vi "Log Data.vi"(0 "Test Inputs":T2 {"Nominal Output Voltage in V" format="%#.5g"; "Load Current in A" format="%#.5g"}, 5 "Test Results":T1 {"Line Regulation in %" format="%#.5g"; "Input Voltage in V" format="%#.5g"; "Input Current in A" format="%#.5g"; "Load Current in A" format="%#.5g"; "Line Regulation in %/V" format="%#.3g"; "Output Voltage in V" format="%#.5g"}, 7 "DataLogger File Path":path, 11 "error in (no error)":errorcluster) -> (15 "error out":errorcluster)   [LabVIEW 2020, in "LDO Line Regulation.lvlib"]
uses:
  LDO Line Regulation.lvlib
  Typedefs/Test Inputs.ctl
  Typedefs/Advance Settings.ctl
  Reusables/Instrument APIs/Load Output Function.ctl
  Typedefs/Test Results.ctl
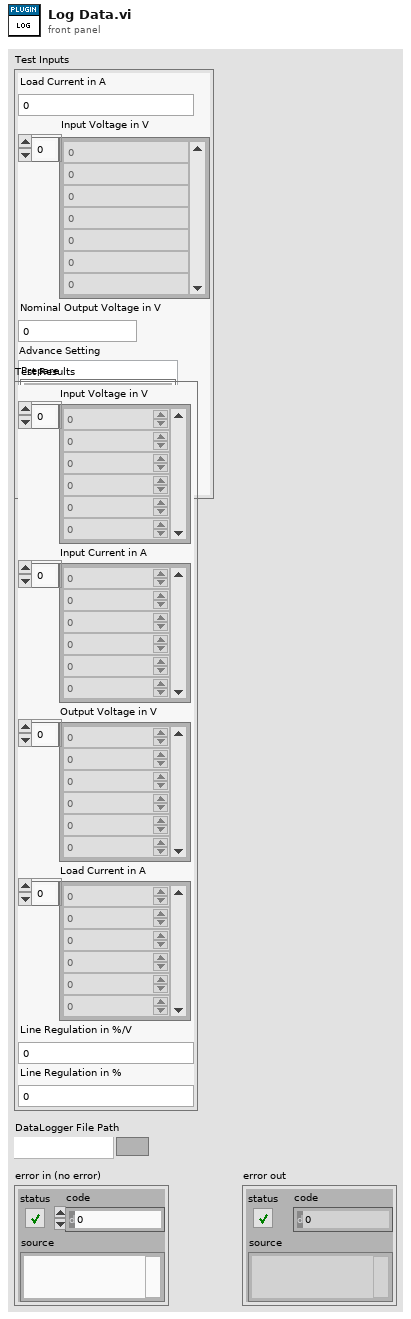
[diagram p1: front panel]
types:
  T1 = typedef "LDO Line Regulation.lvlib/Test Results.ctl" = cluster{"Input Voltage in V":dbl[], "Input Current in A":dbl[], "Output Voltage in V":dbl[], "Load Current in A":dbl[], "Line Regulation in %/V":dbl, "Line Regulation in %":dbl}
  T2 = typedef "LDO Line Regulation.lvlib/Test Inputs.ctl" = cluster{"Load Current in A":dbl, "Input Voltage in V":dbl[], "Nominal Output Voltage in V":dbl, "Advance Setting":T3}
  T3 = typedef "LDO Line Regulation.lvlib/Advance Settings.ctl" = cluster{"Prepare":cluster{"Load SMU Output Function":T4}, "Stimulus And Measure":cluster{"Loop Delay in milliSecond":u32}}
  T4 = typedef "Load Output Function.ctl" = enum16{"VoltageSource", "CurrentSource"}
  T5 = enum16{"open", "replace", "create", "open or create", "replace or create", "replace or create with confirmation"}
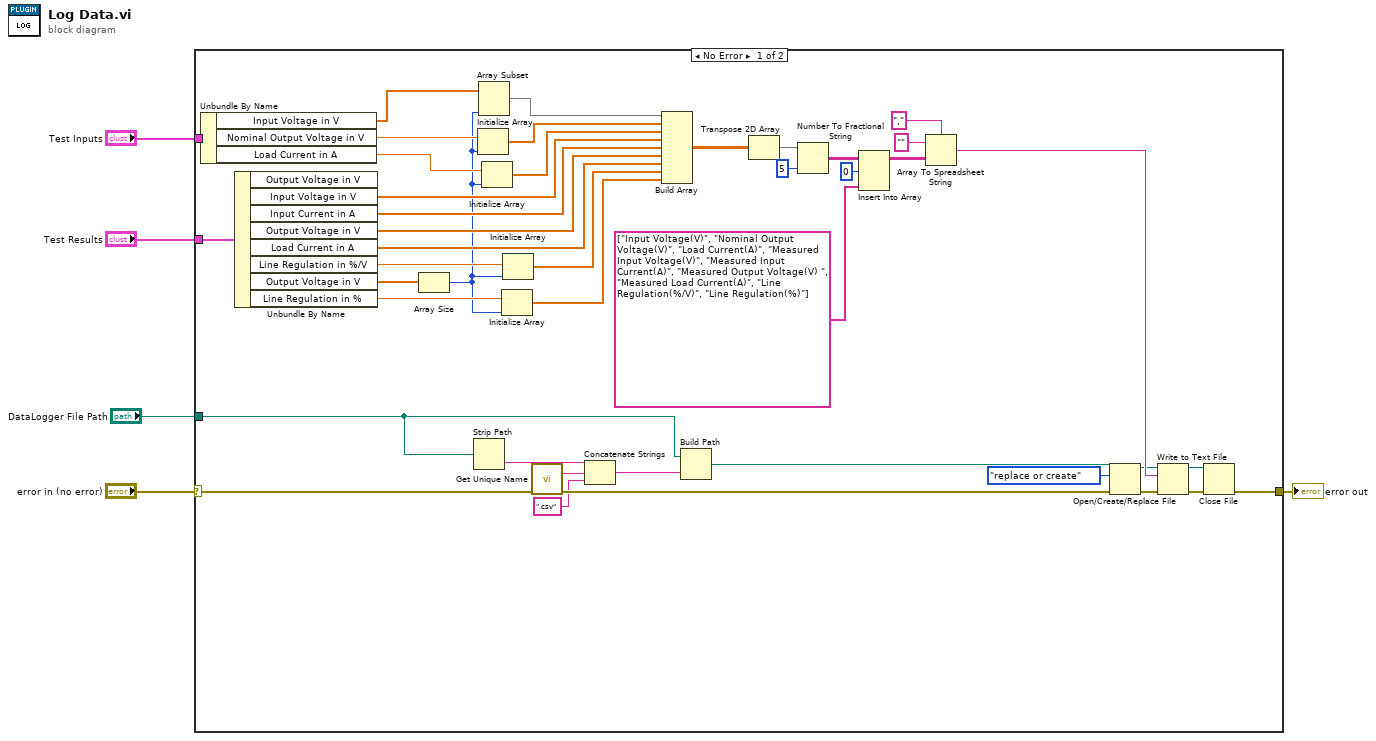
[diagram p0: block diagram]
diagram:
  n1 = case shown="No Error" "error in (no error)" {
    selector: "error in (no error)" -> [w22 w47]
    tunnel: [w30 w47] -> w4
    tunnel: "Test Inputs" -> [w46 _]
    tunnel: "Test Results" -> [w45 _]
    tunnel: "DataLogger File Path" -> [w10 _]
    frame No Error {
      n2 = Unbundle By Name(w46) -> ("Input Voltage in V"=w25:dbl[], "Nominal Output Voltage in V"=w35:dbl, "Load Current in A"=w21:dbl)
      n3 = Unbundle By Name(w45) -> ("Input Voltage in V"=w40:dbl[], "Input Current in A"=w41:dbl[], "Output Voltage in V"=w42:dbl[], "Load Current in A"=w43:dbl[], "Line Regulation in %/V"=w33:dbl, "Output Voltage in V"=w31:dbl[], "Line Regulation in %"=w8:dbl)  [unwired: 1 out]
      n4 = Array Size(array=w31) -> (size(s)=w7:i32)
      n5 = Strip Path(path=w10) -> (name=w13:string)  [unwired: 1 out]
      n6 = Initialize Array(w35, w7) -> (w34:dbl[])
      n7 = Array Subset(array=w25, length=w7) -> (w24:dbl[])  [unwired: 1 in]
      n8 = Initialize Array(w21, w7) -> (w20:dbl[])
      n9 = Initialize Array(w8, w7) -> (w6:dbl[])
      n10 = Initialize Array(w33, w7) -> (w32:dbl[])
      n11 = call "Get Unique Name.vi"() -> ("Unique String"=w14:string)  [unwired: 14 in, 1 out]
      n12 = Concatenate Strings(w13, w14, ".csv" ("format string")) -> (w11:string)
      n13 = Build Array(w24, w34, w20, w40, w41, w42, w43, w32, w6) -> (w39:dbl[][])
      n14 = Build Path(base path=w10, name or relative path=w11) -> (appended path=w9:path)
      n15 = Transpose 2D Array(2D array=w39) -> (transposed array=w44:dbl[][])
      n16 = Number To Fractional String(number=w44, precision (6)=i16 5) -> (F-format string=w36:string[][])  [unwired: 2 in]
      n17 = Insert Into Array(array=w36, index (row)=0, new element=string[] ["Input Voltage(V)", "Nominal Output Voltage(V)", "Load Current(A)", "Measured Input Voltage(V)", "Measured Input Current(A)", "Measured Output Voltage(V) ", "Measured Load Current(A)", "Line Regulation(%/V)", "Line Regulation(%)"] ("new element/subarray")) -> (w27:string[][])  [unwired: 1 in]
      n18 = Array To Spreadsheet String(delimiter (Tab)=",", array=w27, 3:"" ("format string")) -> (spreadsheet string=w26:string)
      n19 = Open/Create/Replace File(file path (use dialog)=w9, error in=w22, operation (0:open)=T5."replace or create") -> (refnum out=w17:refnum<file>, error out=w19:errorcluster)  [unwired: 3 in, 1 out]
      n20 = Write to Text File(file (use dialog)=w17, text=w26, error in=w19) -> (refnum out=w16:refnum<file>, error out=w18:errorcluster)  [unwired: 1 in, 1 out]
      n21 = Close File(refnum=w16, error in=w18) -> (error out=w30:errorcluster)  [unwired: 1 out]
    }
    frame Error {
    }
  }
  "error out" <- w4
